vi "OpenFile.vi"(8 "error in (no error)":errorcluster, 10 "access (0:read/write)":enum16{"read/write", "read-only", "write-only"}(ring), 11 "Path":path) -> (0 "error out":errorcluster, 3 "FileHandler out":refnum<class "FileHandler.lvclass">)   [LabVIEW 2021]
uses:
  Interfaces/FileHandler/FileHandler.lvclass
  Classes/RWFile/RWFile.lvclass
  E:/Programs/LabVIEW/Other Stuff/GLA Summit 2025/LVClassyFile/5. Improvements/Interfaces/FileHandler/FileHandler.lvclass
  Classes/ROFile/ROFile.lvclass
  Classes/WOFile/WOFile.lvclass
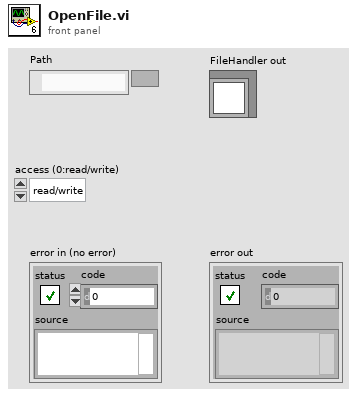
[diagram p1: front panel]
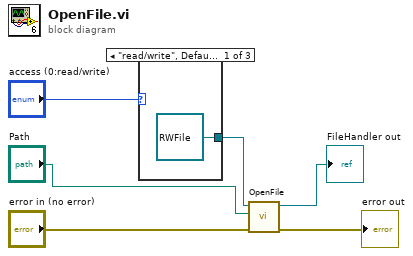
[diagram p0: block diagram]
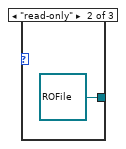
[diagram p2: hidden frame]
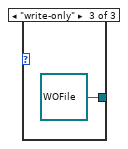
[diagram p3: hidden frame]
diagram:
  n1 = case shown="\"read/write\", Default" "access (0:read/write)" {
    tunnel: [refnum<class "RWFile.lvclass"> refnum ("RWFile.lvclass") refnum<class "ROFile.lvclass"> refnum ("ROFile.lvclass") refnum<class "WOFile.lvclass"> refnum ("WOFile.lvclass")] -> w5
    frame "read/write", Default {
    }
    frame "read-only" {
    }
    frame "write-only" {
    }
  }
  n2 = call-dynamic "OpenFile.vi"("error in (no error)"="error in (no error)", "Path"="Path", "FileHandler in"=w5) -> ("error out"=→"error out":errorcluster, "FileHandler out"=→"FileHandler out":refnum<class "FileHandler.lvclass">)  [unwired: 7 in]
